vi "Selected Items Read.vi"(4 "error in (no error)":errorcluster, 6 "Container State":T2, 7 "Display State In":T1) -> (0 "error out":errorcluster, 2 "Value":string[](array[string]), 3 "Display State Out":T1)   [LabVIEW 2018, in "ListBox XControl.xctl"]
uses:
  ListBox XControl.xctl
  <vilib>/_xctls/Container State.ctl
  State ListBox.ctl
  <vilib>/_xctls/XControlSupport.lvlib
panel:
  # "Replace the Value Indicator below with an Indicator of desired type.\nDo not remove this Indicator or the others from the connector pane. \nDo not change the connector pane pattern.\nThe Value Indicator should always be the second terminal from top on the output side in the connector pane."
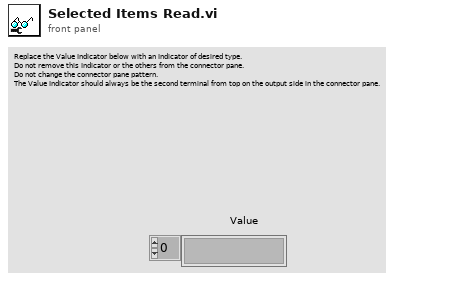
[diagram p1: front panel]
types:
  T1 = typedef "ListBox XControl.xctl/State ListBox.ctl" = cluster{"ItemNames[]":string[], "Listbox Ref":refnum<vi>, "Select All By Default":bool}
  T2 = typedef "XControlSupport.lvlib/Container State.ctl" = cluster{"Indicator?":bool, "Run Mode?":bool, " Refnum":refnum<vi>}
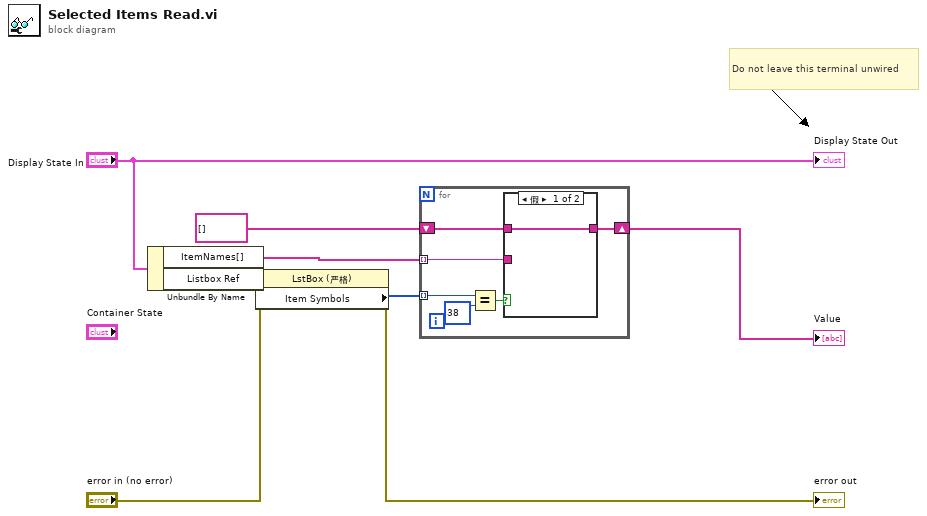
[diagram p0: block diagram]
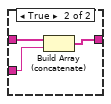
[diagram p2: hidden frame]
diagram:
  # "Do not leave this terminal unwired"
  n1 = Unbundle By Name("Display State In") -> ("ItemNames[]"=w3:string[], "Listbox Ref"=w7:refnum<vi>)
  n2 = property class="LstBox (严格)"(reference=w7, error in="error in (no error)") -> (error out=→"error out":errorcluster, "Item Symbols"=w4:i32[])  [unwired: 1 out]
  n3 = for {
    shift-right: [w9] -> w1
    shift-left: string[] [] ("ItemNames[]") -> [w11]
    tunnel: w4 -> [w14] mode=indexing
    tunnel: w3 -> [w10] mode=indexing
    n4 = Equal?(x=w14, y=38) -> (x = y?=w12:bool)
    n5 = case shown="假" w12 {
      tunnel: w11 -> [w15 w17]
      tunnel: w10 -> [_ w18]
      tunnel: [w15 w16] -> w9
      frame False {
      }
      frame True {
        n6 = Build Array (concatenate)(w17, w18) -> (w16:string[])
      }
    }
  }
  "Value" <- w1
  "Display State Out" <- "Display State In"
